vi "driver_init.vi"() -> (0 "error out":errorcluster, 3 "new reference":refnum<k24>)   [LabVIEW 2021]
uses:
  F:/2PhotonVision/psychometric_function_v2/lib/Grpc.Core.dll
  lib/Grpc.Core.dll
  F:/2PhotonVision/psychometric_function_v2/lib/Grpc.Core.Api.dll
  lib/Grpc.Core.Api.dll
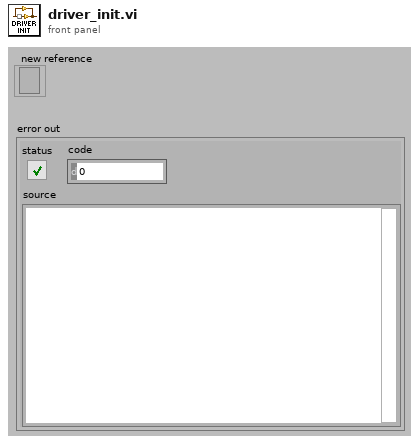
[diagram p1: front panel]
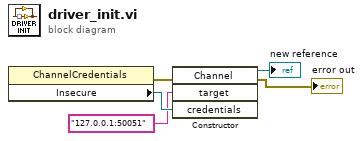
[diagram p0: block diagram]
diagram:
  n1 = property class="ChannelCredentials"() -> (error out=w3:errorcluster, "Insecure"=w5:refnum<k24>)  [unwired: 2 in, 1 out]
  n2 = constructor class="Channel"(error in=w3, "target"="127.0.0.1:50051", "credentials"=w5) -> (reference out=→"new reference":refnum<k24>, error out=→"error out":errorcluster)  [unwired: 2 in, 3 out]
